vi "ml_K Means_Find Nearest Centroids.vi"(10 "Centroids":dbl[][](array[numeric]), 11 "Samples":dbl[][](array[numeric])) -> (1 "nearest centroid":i32[](array[numeric]), 2 "Centroids dup":dbl[][](array[numeric]), 3 "Samples dup":dbl[][](array[numeric]))   [LabVIEW 2013, in "NILabs_MLT.lvlib"]
uses:
  <vilib>/addons/Machine Learning/NILabs_MLT.lvlib
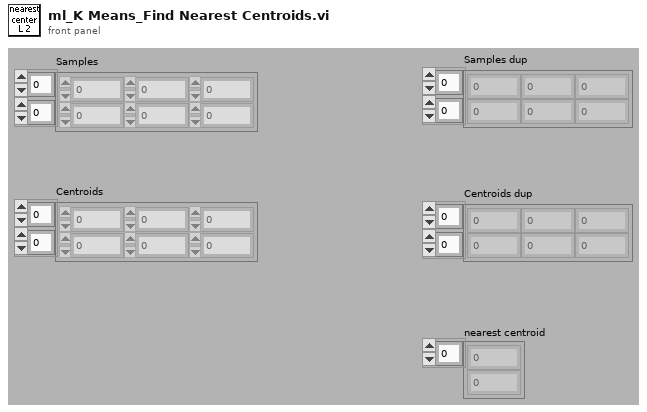
[diagram p1: front panel]
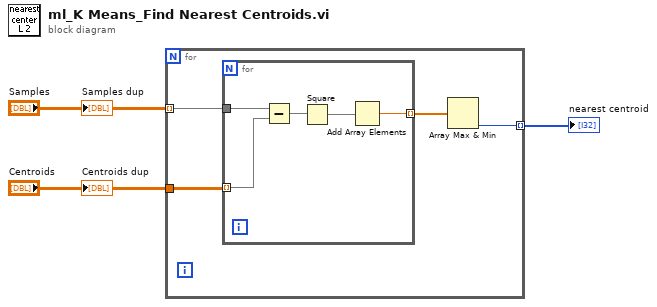
[diagram p0: block diagram]
diagram:
  n1 = for {
    tunnel: "Centroids" -> [w7]
    tunnel: [w5] -> w1 mode=indexing
    tunnel: "Samples" -> [w4] mode=indexing
    n2 = for {
      tunnel: w7 -> [w11] mode=indexing
      tunnel: w4 -> [w12]
      tunnel: [w8] -> w6 mode=indexing
      n3 = Subtract(x=w12, y=w11) -> (x-y=w10:dbl[])
      n4 = Square(x=w10) -> (x^2=w9:dbl[])
      n5 = Add Array Elements(numeric array=w9) -> (sum=w8:dbl)
    }
    n6 = Array Max & Min(array=w6) -> (min index (indices)=w5:i32)  [unwired: 3 out]
  }
  "nearest centroid" <- w1
  "Samples dup" <- "Samples"
  "Centroids dup" <- "Centroids"
